vi "Compass on new GIC C.vi"(11 "GIC Input":T1={"     Use ?\nOff       On"=[FALSE, TRUE, FALSE, TRUE], "Mode:"=FALSE, "Extra Port"="", "Hokuyo Port"="COM7", "Tx Prop  Port"="COM6", "Compass Port"="", "GPS Port"="", "Num of WPs"=0, "WP Lats and Longs"={"WP Lats"=[], "WP Longs"=[]}, "Obst Lats and Longs"={"Obst Lats"=[], "Obst Longs"=[]}, "Parameters"=[], "GPS Data"=[], "Compass"=0.0, "LMS Vector"=[], "Vision Vector"=[], "Direction Cmd"=0.0, "Speed Cmd"=0.0, "WP Vector"=[], "WP Number"=0, "Extra"=0, "SW Map"=[], "Path Cluster"={"Path x node"=[], "Path y node"=[]}, "Sim Course"=[]} {"Obst Lats and Longs"."Obst Longs" format="%#_8g"; "Obst Lats and Longs"."Obst Lats" format="%#_8g"}) -> (3 "GIC Output":T1={"     Use ?\nOff       On"=[FALSE, TRUE, FALSE, TRUE], "Mode:"=FALSE, "Extra Port"="", "Hokuyo Port"="COM7", "Tx Prop  Port"="COM6", "Compass Port"="", "GPS Port"="", "Num of WPs"=0, "WP Lats and Longs"={"WP Lats"=[], "WP Longs"=[]}, "Obst Lats and Longs"={"Obst Lats"=[], "Obst Longs"=[]}, "Parameters"=[], "GPS Data"=[], "Compass"=0.0, "LMS Vector"=[], "Vision Vector"=[], "Direction Cmd"=0.0, "Speed Cmd"=0.0, "WP Vector"=[], "WP Number"=0, "Extra"=0, "SW Map"=[], "Path Cluster"={"Path x node"=[], "Path y node"=[]}, "Sim Course"=[]} {"Obst Lats and Longs"."Obst Longs" format="%#_8g"; "Obst Lats and Longs"."Obst Lats" format="%#_8g"})   [LabVIEW 2014]
panel:
  out "compass out":dbl
  # "Compass on New GIC C"
  # "Input:"
  # "Output:"
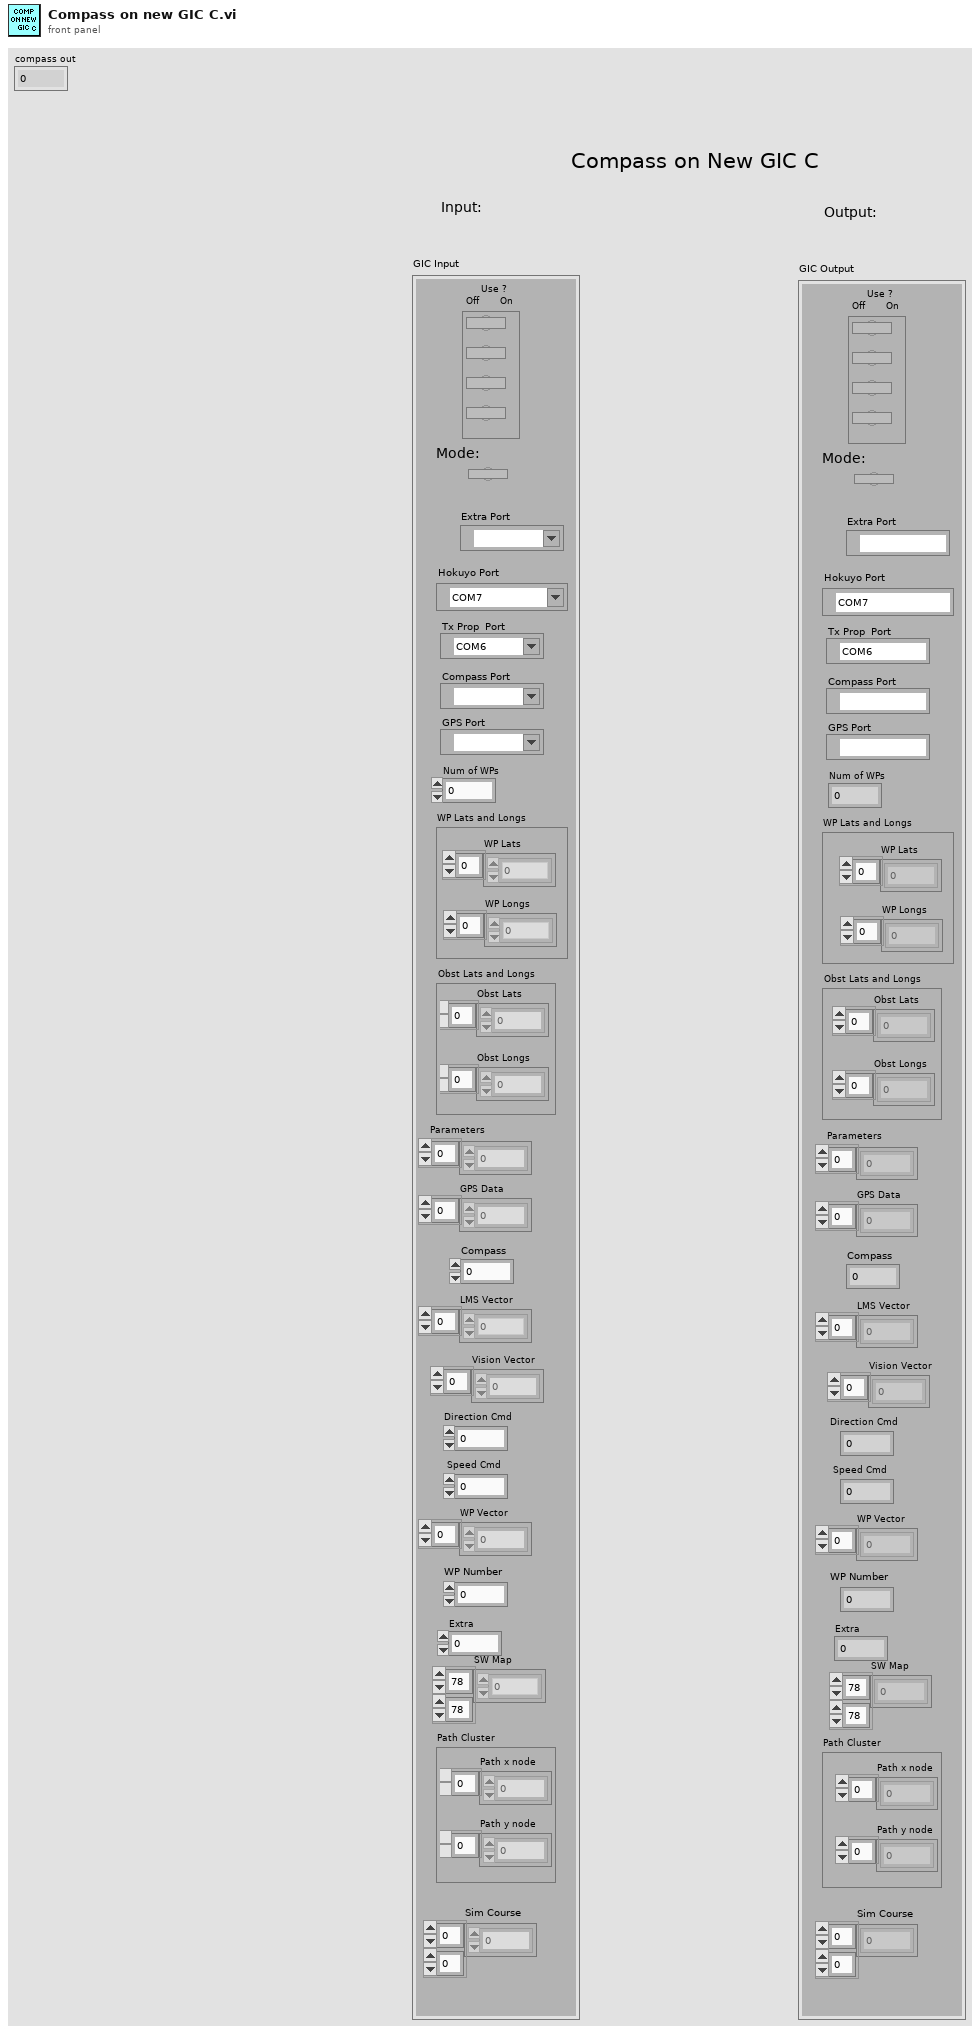
[diagram p1: front panel]
types:
  T1 = cluster{"     Use ?\nOff       On":bool[], "Mode:":bool, "Extra Port":refnum<visa-resource-name>, "Hokuyo Port":refnum<visa-resource-name>, "Tx Prop  Port":refnum<visa-resource-name>, "Compass Port":refnum<visa-resource-name>, "GPS Port":refnum<visa-resource-name>, "Num of WPs":i16, "WP Lats and Longs":cluster{"WP Lats":dbl[], "WP Longs":dbl[]}, "Obst Lats and Longs":cluster{"Obst Lats":dbl[], "Obst Longs":dbl[]}, "Parameters":dbl[], "GPS Data":dbl[], "Compass":dbl, "LMS Vector":dbl[], "Vision Vector":dbl[], "Direction Cmd":dbl, "Speed Cmd":dbl, "WP Vector":dbl[], "WP Number":i32, "Extra":i16, "SW Map":i32[][], "Path Cluster":cluster{"Path x node":dbl[], "Path y node":dbl[]}, "Sim Course":i8[][]}
  T2 = cluster{"     Use ?\nOff       On":bool[], "Mode:":bool, "Rx Prop Port":refnum<visa-resource-name>, "Hokuyo Port":refnum<visa-resource-name>, "Tx Prop  Port":refnum<visa-resource-name>, "Compass Port":refnum<visa-resource-name>, "GPS Port":refnum<visa-resource-name>, "Num of WPs":i16, "WP Lats and Longs":cluster{"WP Lats":dbl[], "WP Longs":dbl[]}, "Obst Lats and Longs":cluster{"Obst Lats":dbl[], "Obst Longs":dbl[]}, "Parameters":dbl[], "GPS Data":dbl[], "Compass":dbl, "LMS Vector":dbl[], "Vision Vector":dbl[], "Direction Cmd":dbl, "Speed Cmd":dbl, "WP Vector":dbl[], "WP Number":i32, "Extra":i16, "SW Map":i32[][], "Path Cluster":cluster{"Path x node":dbl[], "Path y node":dbl[]}, "Sim Course":i8[][]}
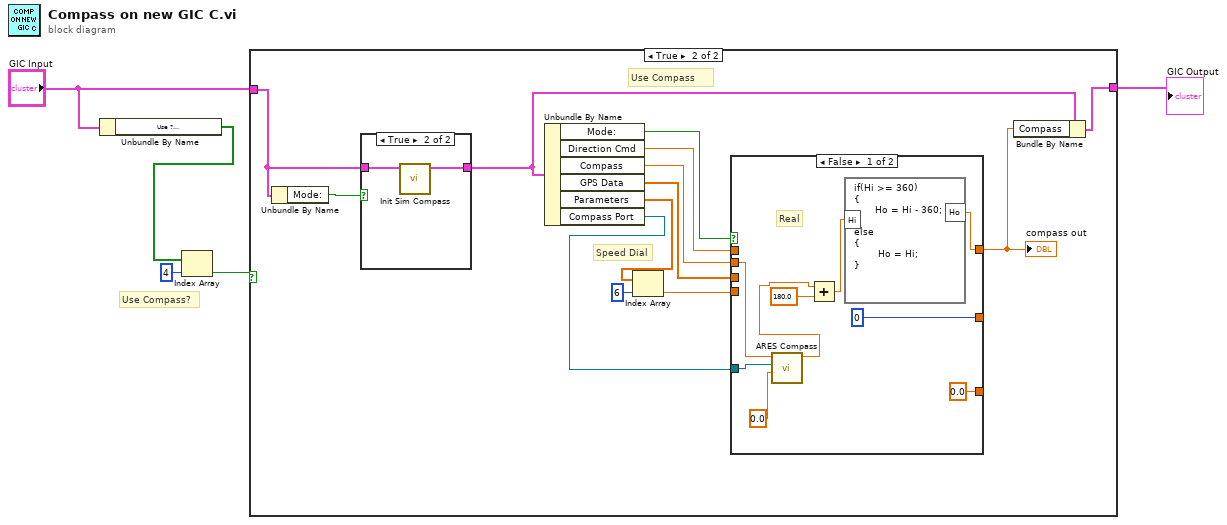
[diagram p0: block diagram]
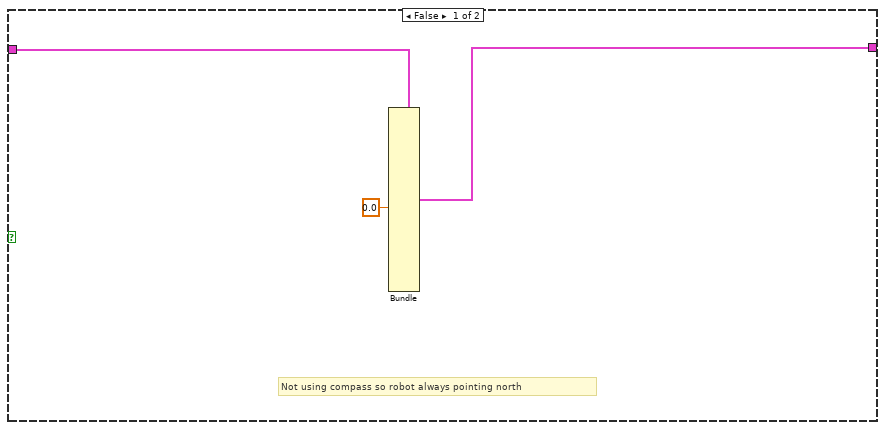
[diagram p2: hidden frame]
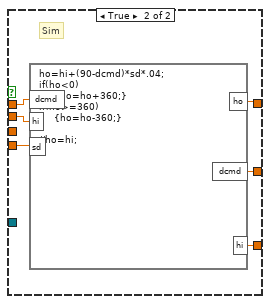
[diagram p4: hidden frame]
diagram:
  # "Use Compass?"
  n1 = Unbundle By Name("GIC Input") -> ("Use ?\nOff       On"=w5:bool[])
  n2 = Index Array(array=w5, index=4) -> (element=w3:bool)
  n3 = case shown="True" w3 {
    tunnel: "GIC Input" -> [w8 w10]
    tunnel: [w6 w16] -> w1
    frame False {
      # "Not using compass so robot always pointing north"
      n4 = Bundle(cluster=w8, "Compass"=0.0) -> (w6:T1)  [unwired: 22 in]
    }
    frame True {
      # "Use Compass"
      # "Speed Dial"
      n5 = Unbundle By Name(w10) -> ("Mode:"=w11:bool)
      n6 = case shown="True" w11 {
        tunnel: w10 -> [w22 w24]
        tunnel: [w22 w23] -> w9
        frame False {
        }
        frame True {
          n7 = call "Init Sim Compass.vi"("GIC Input"=w24) -> ("GIC Output"=w23:T2)  [unwired: 10 in]
        }
      }
      n8 = Unbundle By Name(w9) -> ("Mode:"=w20:bool, "Direction Cmd"=w15:dbl, "Compass"=w14:dbl, "GPS Data"=w21:dbl[], "Parameters"=w19:dbl[], "Compass Port"=w12:refnum<visa-resource-name>)
      n9 = Index Array(array=w19, index=6) -> (element=w17:dbl)
      n10 = case shown="False" w20 {
        tunnel: w15 -> [_ w38]
        tunnel: w14 -> [w31 w37]
        tunnel: [w26 w39] -> w13
        tunnel: w21 -> [_ _]
        tunnel: w17 -> [_ w36]
        tunnel: [0 w35] -> _
        tunnel: [0.0 ("hi") w34] -> _
        tunnel: w12 -> [w30 _]
        frame False {
          # "Real"
          n11 = call "ARES Compass.vi"("Input time of last compass read"=0.0, "Compass Com Port"=w30, "Compass In"=w31) -> ("Compass Out"=w27:dbl)  [unwired: 6 in, 1 out]
          n12 = Add(x=w27, y=180.0) -> (x+y=w25:dbl)
          n13 = formula code="if(Hi >= 360)\n{\n       Ho = Hi - 360;\n}\nelse\n{\n        Ho = Hi;\n}"("Hi"=w25) -> ("Ho"=w26:dbl)
        }
        frame True {
          # "Sim"
          n14 = formula code="ho=hi+(90-dcmd)*sd*.04;\nif(ho<0)\n     {ho=ho+360;}\nif(ho>=360)\n     {ho=ho-360;}\n\n//ho=hi;"("dcmd"=w38, "hi"=w37, "sd"=w36) -> ("ho"=w39:dbl, "dcmd"=w35:dbl, "hi"=w34:dbl)
        }
      }
      "compass out" <- w13
      n15 = Bundle By Name(cluster=w9, "Compass"=w13) -> (w16:T2)
    }
  }
  "GIC Output" <- w1
